vi "ValidacaoOndaSenoide.vi"(11 "InfoInSenoide":T1={"Texpontos senoide"="O máximo é 60 pontos por minuto", "PicoRotacaoMax"=0.0, "PicoRotacaoMin"=0.0, "RotaçõesMinuto"=0.0, "PontosMinuto"=0.0}) -> (0 "error out":errorcluster)   [LabVIEW 2019]
uses:
  TelaConfig/Configuracao.Variaveis.vi
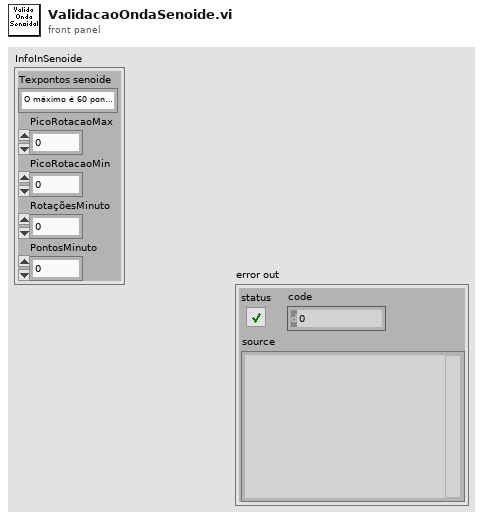
[diagram p1: front panel]
types:
  T1 = cluster{"Texpontos senoide":string, "PicoRotacaoMax":dbl, "PicoRotacaoMin":dbl, "RotaçõesMinuto":dbl, "PontosMinuto":dbl}
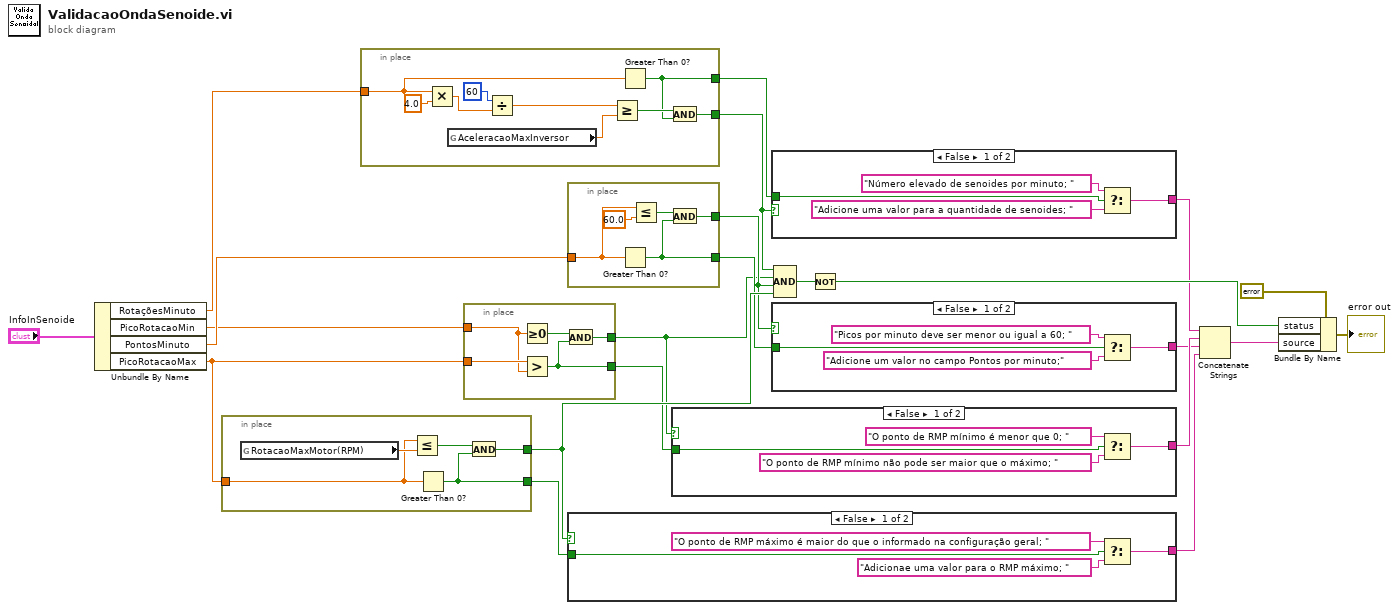
[diagram p0: block diagram]
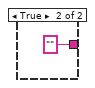
[diagram p2: hidden frame]
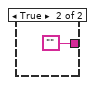
[diagram p3: hidden frame]
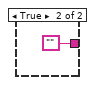
[diagram p4: hidden frame]
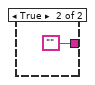
[diagram p5: hidden frame]
diagram:
  n1 = Unbundle By Name("InfoInSenoide") -> ("RotaçõesMinuto"=w6:dbl, "PicoRotacaoMin"=w3:dbl, "PontosMinuto"=w4:dbl, "PicoRotacaoMax"=w5:dbl)
  n2 = in-place {
    in-place-border: [w25] -> w10
    in-place-border: [w24] -> w9
    in-place-border: w5 -> [w23]
    n3 = global read "Configuracao.Variaveis.vi" "RotacaoMaxMotor(RPM)"() -> (w27:dbl)
    n4 = Less Or Equal?(x=w23, y=w27) -> (x <= y?=w26:bool)
    n5 = Greater Than 0?(x=w23) -> (x > 0?=w24:bool)
    n6 = And(x=w26, y=w24) -> (x .and. y?=w25:bool)
  }
  n7 = in-place {
    in-place-border: [w30] -> w12
    in-place-border: [w29] -> w11
    in-place-border: w6 -> [w28]
    n8 = Multiply(x=w28, y=4.0) -> (x*y=w34:dbl)
    n9 = global read "Configuracao.Variaveis.vi" "AceleracaoMaxInversor"() -> (w32:dbl)
    n10 = Divide(x=60, y=w34) -> (x/y=w33:dbl)
    n11 = Greater Or Equal?(x=w33, y=w32) -> (x >= y?=w31:bool)
    n12 = Greater Than 0?(x=w28) -> (x > 0?=w29:bool)
    n13 = And(x=w31, y=w29) -> (x .and. y?=w30:bool)
  }
  n14 = in-place {
    in-place-border: w5 -> [w41]
    in-place-border: w3 -> [w40]
    in-place-border: [w38] -> w2
    in-place-border: [w37] -> w1
    n15 = Greater Or Equal To 0?(x=w40) -> (x >= 0?=w39:bool)
    n16 = Greater?(x=w41, y=w40) -> (0:w37:bool)
    n17 = And(x=w39, y=w37) -> (x .and. y?=w38:bool)
  }
  n18 = in-place {
    in-place-border: [w45] -> w8
    in-place-border: [w44] -> w7
    in-place-border: w4 -> [w42]
    n19 = Greater Than 0?(x=w42) -> (x > 0?=w45:bool)
    n20 = Less Or Equal?(x=w42, y=60.0) -> (x <= y?=w43:bool)
    n21 = And(x=w43, y=w45) -> (x .and. y?=w44:bool)
  }
  n22 = case shown="False" w10 {
    tunnel: [w50 ""] -> w13
    tunnel: w9 -> [w49 _]
    frame False {
      n23 = Select(t="O ponto de RMP máximo é maior do que o informado na configuração geral; ", s=w49, f="Adicionae uma valor para o RMP máximo; ") -> (s? t:f=w50:string)
    }
    frame True {
    }
  }
  n24 = case shown="False" w2 {
    tunnel: [w52 ""] -> w15
    tunnel: w1 -> [w55 _]
    frame False {
      n25 = Select(t="O ponto de RMP mínimo é menor que 0; ", s=w55, f="O ponto de RMP mínimo não pode ser maior que o máximo; ") -> (s? t:f=w52:string)
    }
    frame True {
    }
  }
  n26 = case shown="False" w12 {
    tunnel: [w59 ""] -> w16
    tunnel: w11 -> [w60 _]
    frame False {
      n27 = Select(t="Número elevado de senoides por minuto; ", s=w60, f="Adicione uma valor para a quantidade de senoides; ") -> (s? t:f=w59:string)
    }
    frame True {
    }
  }
  n28 = case shown="False" w7 {
    tunnel: [w64 ""] -> w14
    tunnel: w8 -> [w63 _]
    frame False {
      n29 = Select(t="Picos por minuto deve ser menor ou igual a 60; ", s=w63, f="Adicione um valor no campo Pontos por minuto;") -> (s? t:f=w64:string)
    }
    frame True {
    }
  }
  n30 = Compound Arithmetic op=AND(w12, w2, w7, w10) -> (w18:bool)
  n31 = Not(x=w18) -> (.not. x?=w17:bool)
  n32 = Concatenate Strings(w16, w15, w14, w13) -> (w20:string)
  n33 = Bundle By Name(cluster=errorcluster {"status"=FALSE, "code"=0, "source"=""} ("error out"), "status"=w17, "source"=w20) -> (→"error out":errorcluster)
